vi "Fundamental Vector.vi"(0 "waveforms":waveform(dbl)[](array[waveform]), 9 "system info in":refnum<class "EP System Info.lvclass">, 11 "error in (no error)":errorcluster) -> (4 "one-cycle fundamental vectors":T2(array[cluster]), 10 "system info out":refnum<class "EP System Info.lvclass">, 15 "error out":errorcluster)   [LabVIEW 2014, in "NI_EP_Power Quality.lvlib"]
doc: "Calculates the fundamental vector for each cycle contained in the input waveforms.\n\nThis VI supports measuring single-line and multiple-line systems."
uses:
  <vilib>/addons/Electrical Power/PQ/NI_EP_Power Quality.lvlib
  <vilib>/addons/Electrical Power/PQ/Common/Controls/ep_AI Data Channel.ctl
  <vilib>/addons/Electrical Power/PQ/Common/Classes/System Info/EP System Info.lvclass
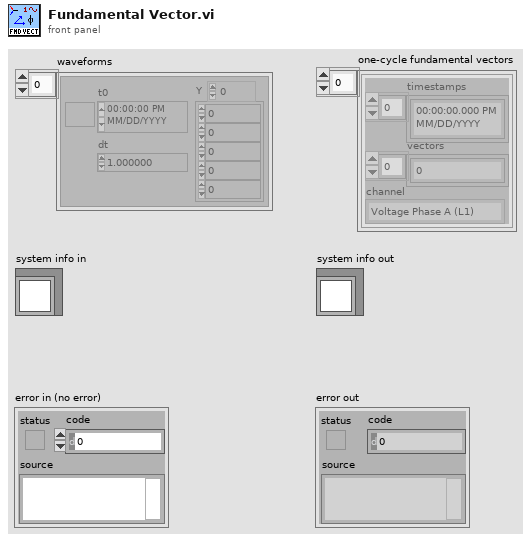
[diagram p1: front panel]
types:
  T1 = typedef "NI_EP_Power Quality.lvlib/ep_AI Data Channel.ctl" = enum16{"Voltage Phase A (L1)", "Voltage Phase B (L2)", "Voltage Phase C (L3)", "Voltage Phase N (Neutral)", "Current Phase A (L1)", "Current Phase B (L2)", "Current Phase C (L3)", "Current Phase N (Neutral)"}
  T2 = cluster{"timestamps":timestamp[], "vectors":cdb[], "channel":T1}[]
  T3 = cluster{timestamp[], cdb[], "AI data channel":T1}
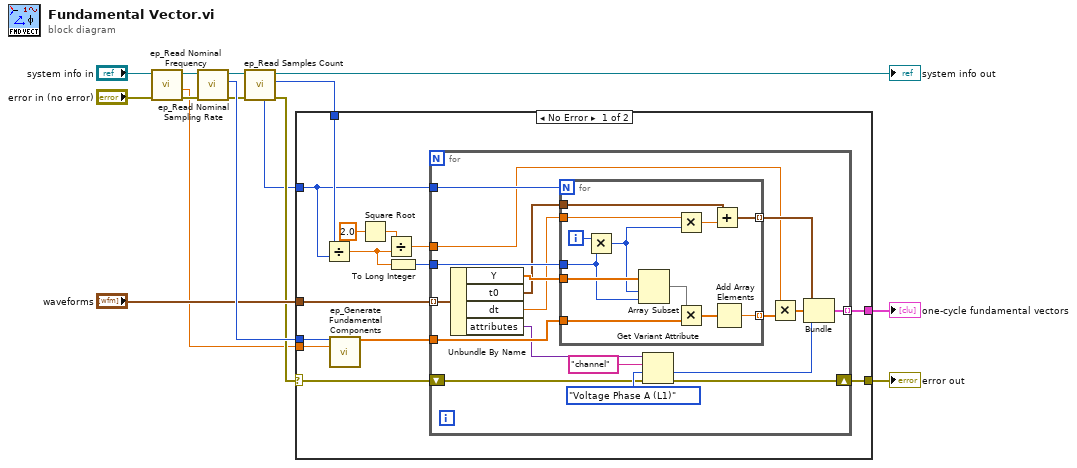
[diagram p0: block diagram]
diagram:
  n1 = call <vilib>:"ep_Read Nominal Frequency.vi"("error in (no error)"="error in (no error)", "system info in"="system info in") -> ("error out"=w13:errorcluster, "nominal frequency value"=w2:dbl, "system info out"=w15:refnum<class "EP System Info.lvclass">)  [unwired: 6 in, 1 out]
  n2 = call <vilib>:"ep_Read Nominal Sampling Rate.vi"("error in (no error)"=w13, "system info in"=w15) -> ("error out"=w7:errorcluster, "nominal sampling rate (Hz)"=w11:u16, "system info out"=w9:refnum<class "EP System Info.lvclass">)  [unwired: 7 in]
  n3 = call <vilib>:"ep_Read Samples Count.vi"("error in (no error)"=w7, "system info in"=w9) -> ("error out"=w4:errorcluster, "basic calc. interval (samples)"=w5:i32, "system info out"=→"system info out":refnum<class "EP System Info.lvclass">, "cycles per interval"=w3:i32)  [unwired: 5 in, 1 out]
  n4 = case shown="No Error" w4 {
    selector: w4 -> [w17 w60]
    tunnel: w11 -> [w29 _]
    tunnel: "waveforms" -> [w28 _]
    tunnel: [w21 _] -> w6
    tunnel: w5 -> [w20 _]
    tunnel: w2 -> [w19 _]
    tunnel: w3 -> [w18 _]
    tunnel: [w16 w60] -> w1
    frame No Error {
      n5 = Divide(x=w20, y=w18) -> (x/y=w24:dbl)
      n6 = call <vilib>:"ep_Generate Fundamental Components.vi"("nominal sampling rate (Hz)"=w29, "nominal frequency value"=w19) -> ("cos - j*sin"=w22:cdb[])  [unwired: 13 in]
      n7 = Square Root(x=2.0) -> (sqrt(x)=w27:dbl)
      n8 = Divide(x=w27, y=w24) -> (x/y=w25:dbl)
      n9 = To Long Integer(number=w24) -> (32bit integer=w23:i32)
      n10 = for {
        tunnel: w18 -> [w45]
        tunnel: w28 -> [w46] mode=indexing
        tunnel: w25 -> [w36]
        tunnel: w23 -> [w44]
        tunnel: w22 -> [w43]
        tunnel: [w42] -> w21 mode=indexing
        shift-right: [w30] -> w16
        shift-left: w17 -> [w31]
        n11 = Unbundle By Name(w46) -> ("Y"=w47:dbl[], "t0"=w40:timestamp, "dt"=w41:dbl, "attributes"=w34:variant)
        n12 = for {
          N: w45 -> [_]
          tunnel: w47 -> [w59]
          tunnel: w43 -> [w56]
          tunnel: [w51] -> w37 mode=indexing
          tunnel: w44 -> [w49]
          tunnel: w41 -> [w55]
          tunnel: w40 -> [w53]
          tunnel: [w52] -> w39 mode=indexing
          i -> [w58]
          n13 = Multiply(x=w58, y=w49) -> (x*y=w48:i32)
          n14 = Array Subset(array=w59, index=w48, length=w49) -> (w50:dbl[])
          n15 = Multiply(x=w55, y=w48) -> (x*y=w54:dbl)
          n16 = Multiply(x=w50, y=w56) -> (x*y=w57:cdb[])
          n17 = Add(x=w53, y=w54) -> (x+y=w52:timestamp)
          n18 = Add Array Elements(numeric array=w57) -> (sum=w51:cdb)
        }
        n19 = Get Variant Attribute(Variant=w34, name="channel", default value (empty Variant)=ep_AI_Data_Channel."Voltage Phase A (L1)" ("AI data channel"), error in=w31) -> (value=w32:T1, error out=w30:errorcluster)  [unwired: 2 out]
        n20 = Multiply(x=w36, y=w37) -> (x*y=w38:cdb[])
        n21 = Bundle(w39, w38, "AI data channel"=w32) -> (w42:T3)  [unwired: 1 in]
      }
    }
    frame Error {
    }
  }
  "error out" <- w1
  "one-cycle fundamental vectors" <- w6
